vi "Read Frequency Scan Point.vi"(8 "error in (no error)":errorcluster, 10 "additional timeout, ms (0)":u32, 11 "VI Probe in":refnum<class "PL MKS VI Probe.lvclass">) -> (0 "error out":errorcluster, 1 "end of scan":bool, 2 "scan point":T1, 3 "VI Probe out":refnum<class "PL MKS VI Probe.lvclass">)   [LabVIEW 2015, in "PL MKS VI Probe.lvclass"]
doc: "Reads frequency scan point. If <b>end of scan</b> is true, point data is not valid."
uses:
  PL MKS VI Probe.lvclass
  PL MKS VI Probe.lvclass/PL MKS VI Probe.ctl
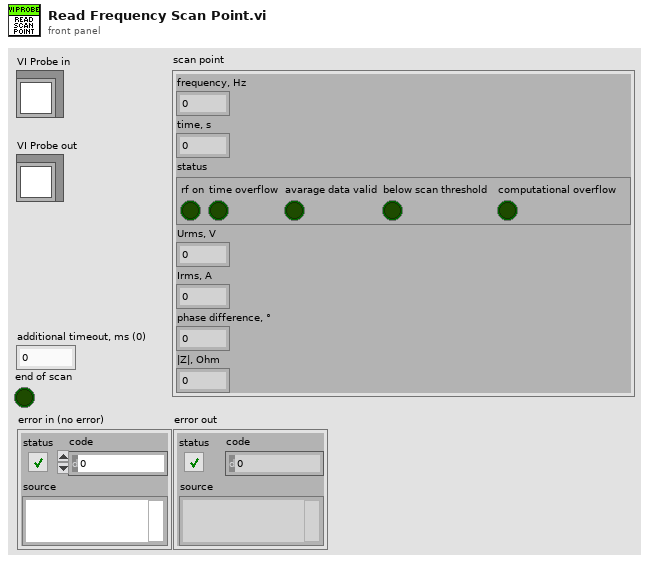
[diagram p1: front panel]
types:
  T1 = cluster{"frequency, Hz":u32, "time, s":dbl, "status":cluster{"rf on":bool, "time overflow":bool, "avarage data valid":bool, "below scan threshold":bool, "computational overflow":bool}, "Urms, V":dbl, "Irms, A":dbl, "phase difference, °":dbl, "|Z|, Ohm":dbl}
  T2 = cluster{"[0]":bool, "[1]":bool, "[2]":bool, "[3]":bool, "[4]":bool}
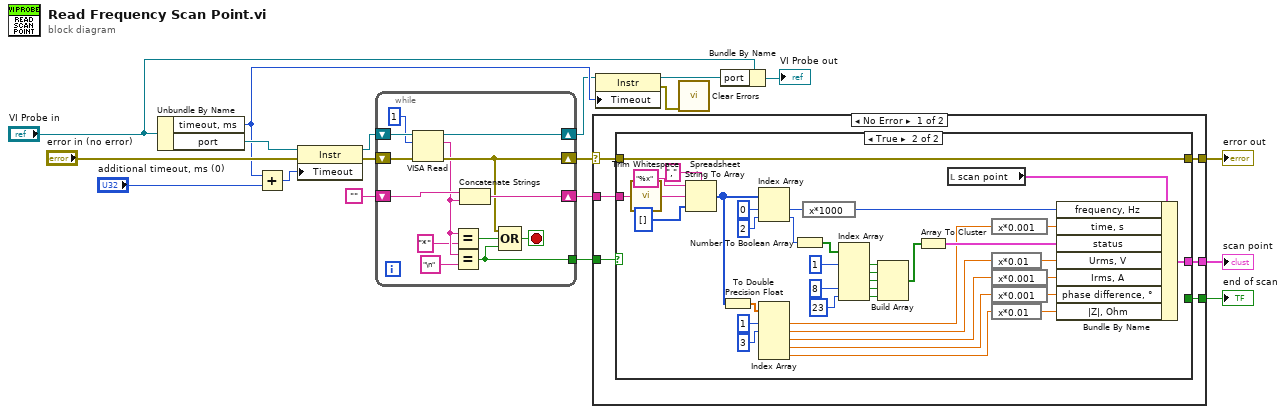
[diagram p0: block diagram]
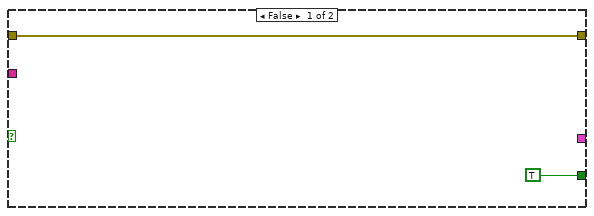
[diagram p2: hidden frame]
diagram:
  n1 = Unbundle By Name("VI Probe in") -> ("timeout, ms"=w11:u32, "port"=w16:refnum<visa-resource-name>)
  n2 = Add(x=w11, y="additional timeout, ms (0)") -> (x+y=w14:u32)
  n3 = property class="Instr"(reference=w16, error in="error in (no error)", "Timeout"=w14) -> (reference out=w12:refnum<visa-resource-name>, error out=w13:errorcluster)
  n4 = while {
    shift-right: [w25] -> w5
    shift-left: w13 -> [w31]
    shift-right: [w30] -> w2
    shift-left: w12 -> [w32]
    shift-right: [w28] -> w3
    shift-left: "" -> [w27]
    tunnel: [w20] -> w4
    stop <- w26 stop-if-true
    n5 = VISA Read(VISA resource name=w32, byte count=u32 1, error in (no error)=w31) -> (VISA resource name out=w30:refnum<visa-resource-name>, read buffer=w23:string, error out=w25:errorcluster)  [unwired: 1 out]
    n6 = Equal?(x=w23, y="*") -> (x = y?=w24:bool)
    n7 = Equal?(x=w23, y="\n") -> (x = y?=w20:bool)
    n8 = Concatenate Strings(w27, w23) -> (w28:string)
    n9 = Compound Arithmetic op=OR(w25, w24, w20) -> (w26:bool)
  }
  n10 = case shown="No Error" w5 {
    selector: w5 -> [w37 w79]
    tunnel: [w36 w79] -> w8
    tunnel: w4 -> [w33 _]
    tunnel: w3 -> [w38 _]
    tunnel: [w35 _] -> w1
    tunnel: [w34 _] -> w7
    frame No Error {
      n11 = case shown="True" w33 {
        tunnel: w38 -> [_ w78]
        tunnel: w37 -> [w40 w64]
        tunnel: [w40 w64] -> w36
        tunnel: [_ w42] -> w35
        tunnel: [TRUE ("end of scan") _] -> w34
        frame False {
        }
        frame True {
          n12 = call <vilib>:"Trim Whitespace.vi"("string"=w78) -> ("trimmed string"=w77:string)  [unwired: 1 in]
          n13 = Spreadsheet String To Array(delimiter (Tab)=",", format string="%x", spreadsheet string=w77, array type (2D Dbl)=u32[] []) -> (array=w69:u32[])
          n14 = To Double Precision Float(number=w69) -> (double precision float=w68:dbl[])
          n15 = Index Array(array=w69, index #1=0 ("index"), index #2=2 ("index")) -> (element #1=w67:u32, element #2=w65:u32)
          n16 = Index Array(array=w68, index #1=1 ("index"), index #2=3 ("index")) -> (element #1=w52:dbl, element #2=w51:dbl, element #3=w50:dbl, element #4=w49:dbl, element #5=w48:dbl)  [unwired: 3 in]
          n17 = Number To Boolean Array(number=w65) -> (Boolean array=w60:bool[])
          n18 = expression code="x*1000"(w67) -> (w66:u32)
          n19 = Index Array(array=w60, index #1=1 ("index"), index #4=8 ("index"), index #5=23 ("index")) -> (element #1=w59:bool, element #2=w55:bool, element #3=w56:bool, element #4=w57:bool, element #5=w58:bool)  [unwired: 2 in]
          n20 = Build Array(w59, w55, w56, w57, w58) -> (w54:bool[])
          n21 = Array To Cluster(array=w54) -> (cluster=w53:T2)
          n22 = local read "scan point"() -> (w41:T1)
          n23 = expression code="x*0.001"(w52) -> (w47:dbl)
          n24 = expression code="x*0.01"(w51) -> (w46:dbl)
          n25 = expression code="x*0.001"(w50) -> (w45:dbl)
          n26 = expression code="x*0.001"(w49) -> (w44:dbl)
          n27 = expression code="x*0.01"(w48) -> (w43:dbl)
          n28 = Bundle By Name(cluster=w41, "frequency, Hz"=w66, "time, s"=w47, "status"=w53, "Urms, V"=w46, "Irms, A"=w45, "phase difference, °"=w44, "|Z|, Ohm"=w43) -> (w42:T1)
        }
      }
    }
    frame Error {
    }
  }
  "error out" <- w8
  "end of scan" <- w7
  "scan point" <- w1
  n29 = property class="Instr"(reference=w2, "Timeout"=w11) -> (reference out=w10:refnum<visa-resource-name>, error out=w9:errorcluster)  [unwired: 1 in]
  n30 = call <vilib>:"Clear Errors.vi"("error in (no error)"=w9) -> ()  [unwired: 5 in, 2 out]
  n31 = Bundle By Name(cluster="VI Probe in", "port"=w10) -> (→"VI Probe out":refnum<class "PL MKS VI Probe.lvclass">)
